vi "Rectangle bounds to size.vi"(11 "bounds":T2 {"bottom" format="%.3f"; "right" format="%.3f"; "top" format="%.3f"; "left" format="%.3f"}) -> (0 "bounds at 0,0 origin":T2 {"bottom" format="%.3f"; "right" format="%.3f"; "top" format="%.3f"; "left" format="%.3f"}, 1 "height":dbl format="%.3f", 2 "width":dbl format="%.3f", 3 "size":T1 {"Y" format="%.3f"; "X" format="%.3f"}, 4 "left top":T1 {"Y" format="%.3f"; "X" format="%.3f"})   [LabVIEW 2023]
doc: "LTRB bounds to Width and Height"
uses:
  Controls/Rect or Line Cluster.ctl
  Controls/x,y cluster_DBL.ctl
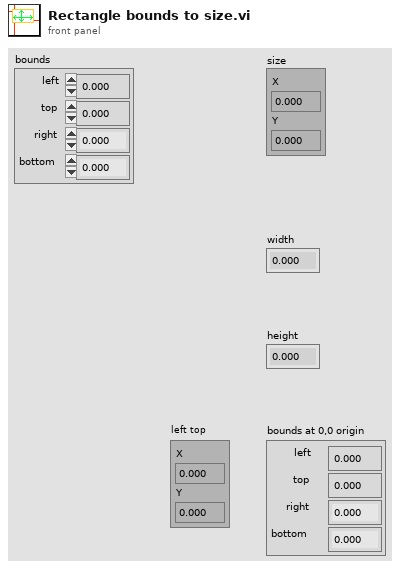
[diagram p1: front panel]
types:
  T1 = typedef "x,y cluster_DBL.ctl" = cluster{"X":dbl, "Y":dbl}
  T2 = typedef "Rect or Line Cluster.ctl" = cluster{"left":dbl, "top":dbl, "right":dbl, "bottom":dbl}
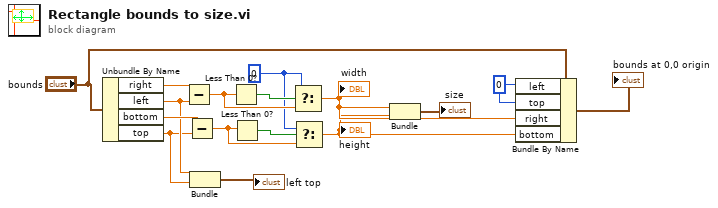
[diagram p0: block diagram]
diagram:
  w5 = 0
  w13 = i16 0 ("Left")
  n1 = Unbundle By Name("bounds") -> ("right"=w16:dbl, "left"=w3:dbl, "bottom"=w15:dbl, "top"=w2:dbl)
  n2 = Subtract(x=w16, y=w3) -> (x-y=w9:dbl)
  n3 = Subtract(x=w15, y=w2) -> (x-y=w6:dbl)
  n4 = Bundle("left"=w3, "top"=w2) -> (→"left top":cluster{"left":dbl, "top":dbl})  [unwired: 1 in]
  n5 = Less Than 0?(x=w9) -> (x < 0?=w10:bool)
  n6 = Less Than 0?(x=w6) -> (x < 0?=w7:bool)
  n7 = Select(t=w5, s=w10, f=w9) -> (s? t:f=w8:dbl)
  "width" <- w8
  n8 = Select(t=w5, s=w7, f=w6) -> (s? t:f=w4:dbl)
  "height" <- w4
  n9 = Bundle(w8, w4) -> (→"size":cluster{dbl, dbl})  [unwired: 1 in]
  n10 = Bundle By Name(cluster="bounds", "left"=w13, "top"=w13, "right"=w8, "bottom"=w4) -> (→"bounds at 0,0 origin":T2)
